vi "MB Ethernet Master Query Read Holding Registers (poly).vi"(0 "TCP Connection Refnum in":refnum<k5>, 1 "Starting Address":u16, 2 "Quantity":u16, 4 "Timeout":u32=10000, 5 "error in":errorcluster, 6 "MBAP Header":cluster{"Transaction ID":u16, "Unit ID":u8}) -> (14 "TCP Connection Refnum (dup)":refnum<k5>, 15 "Holding Registers":u16[](array[numeric]), 16 "Exception Code":u8 format="%.0x", 19 "error out":errorcluster)   [LabVIEW 2011]
doc: "The master uses this VI to read the slaves' holding registers. This corresponds to a public function code of 3 in the MODBUS protocol."
uses:
  MB Modbus Command.ctl
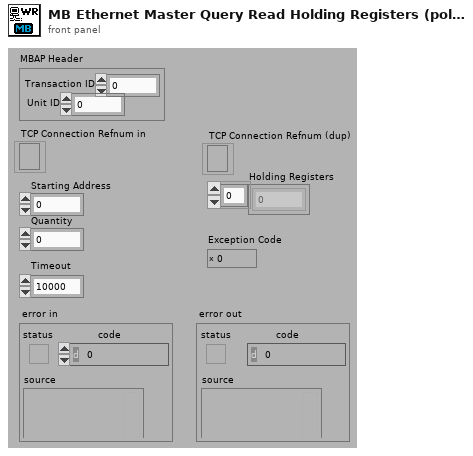
[diagram p1: front panel]
types:
  T1 = typedef "MB Modbus Command.ctl" = cluster{"Function Code":u8, "Starting Address":u16, "Quantity":u16, "Data":u16[], "Discrete":bool[]}
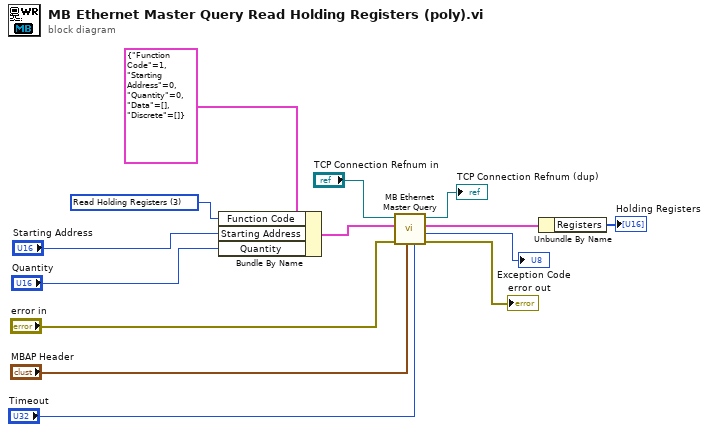
[diagram p0: block diagram]
diagram:
  w12 = u8 3 items=["Read Coils"=1, "Read Discrete Inputs"=2, "Read Holding Registers"=3, "Read Input Registers"=4, "Write Single Coil"=5, "Write Single Register"=6, "Read Exception Status"=7, "Write Multiple Coils"=15, "Write Multiple Registers"=16] ("Function Code")
  n1 = Bundle By Name(cluster=T1 {"Function Code"=1, "Starting Address"=0, "Quantity"=0, "Data"=[], "Discrete"=[]} ("Modbus Command"), "Function Code"=w12, "Starting Address"="Starting Address", "Quantity"="Quantity") -> (w13:T1)
  n2 = call "MB Ethernet Master Query.vi"("Timeout"="Timeout", "MBAP Header"="MBAP Header", "error in (no error)"="error in", "Modbus Command"=w13, "TCP Connection Refnum in"="TCP Connection Refnum in") -> ("error out"=→"error out":errorcluster, "Exception Code"=→"Exception Code":u8, "Registers"=w5:cluster{"Registers":u16[], "Discrete":bool[]}, "TCP Connection Refnum (dup)"=→"TCP Connection Refnum (dup)":refnum<k5>)  [unwired: 2 in, 1 out]
  n3 = Unbundle By Name(w5) -> ("Registers"=→"Holding Registers":u16[])
